vi "Test Handle Help.vi"(11 "Instrument in":refnum<class "Instrument.lvclass">) -> (2 "Array":variant[](array[variant]), 3 "Instrument out":refnum<class "Instrument.lvclass">, 8 "error out":errorcluster)   [LabVIEW 2019, in "Instrument.lvclass"]
uses:
  Instrument.lvclass
  Instrument Types/Strain/Instrument.Strain.lvclass
  C:/Users/patrick/Documents/GitHub/Instrument-Framework/lvsrc/Framework/Instrument/Instrument.lvclass
panel:
  in  "error in (no error)":errorcluster
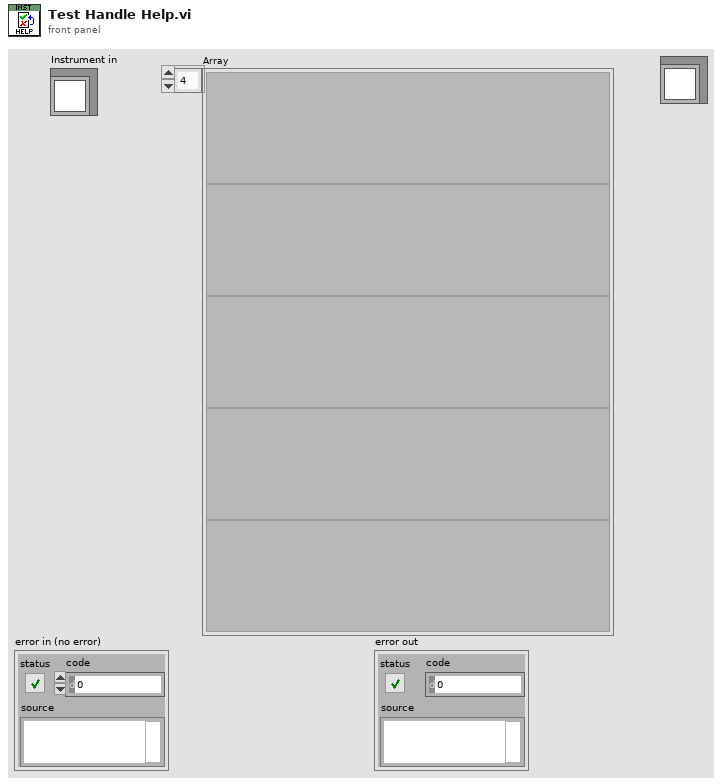
[diagram p1: front panel]
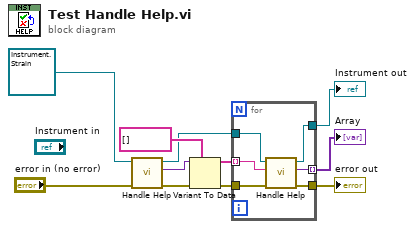
[diagram p0: block diagram]
diagram:
  n1 = call "Handle Help.vi"("error in (no error)"="error in (no error)", "Instrument in"=refnum<class "Instrument.Strain.lvclass"> refnum ("Instrument.Strain.lvclass")) -> ("error out"=w5:errorcluster, "Help"=w11:variant, "Instrument out"=w9:refnum<class "Instrument.Strain.lvclass">)  [unwired: 7 in]
  n2 = Variant To Data(error in=w5, type=string[] [], Variant=w11) -> (data=w8:string[], error out=w4:errorcluster)
  n3 = for {
    tunnel: w9 -> [w17]
    tunnel: w8 -> [w16] mode=indexing
    tunnel: [w15] -> w7 mode=indexing
    tunnel: [w14] -> w6
    tunnel: w4 -> [w13]
    tunnel: [w12] -> w3
    n4 = call "Handle Help.vi"("error in (no error)"=w13, "Command"=w16, "Instrument in"=w17) -> ("error out"=w12:errorcluster, "Help"=w15:variant, "Instrument out"=w14:refnum<class "Instrument.Strain.lvclass">)  [unwired: 6 in]
  }
  "Array" <- w7
  "Instrument out" <- w6
  "error out" <- w3
